vi "Avoid Obstacle with Unicycle Model.vi"(9 "V forward":dbl, 10 "Posture In":dbl[](array[numeric]), 11 "IF readings\n(meters)":dbl[](array[numeric]) format="%_6g") -> (3 "Frame Velocity":dbl[](array[numeric]))   [LabVIEW 2016]
uses:
  <vilib>/Analysis/coordinate.llb/Angle Range (Degree).ctl
  <vilib>/Analysis/coordinate.llb/Angle Units.ctl
  <vilib>/Analysis/coordinate.llb/Wrap Angle (scalar).vi
  <vilib>/Analysis/NI_AAL_Angle.lvlib
panel:
  in  "K Gain":dbl=12.0
  out "atan2(y,x)":dbl
  out "x-y":dbl
  out "output":dbl format="%.2f"
  in  "Sensor Gain":dbl[](array[numeric])=[1.0, 1.0, 0.5, 1.0, 1.0]
  out "ir distances wf":dbl[][](array[numeric])
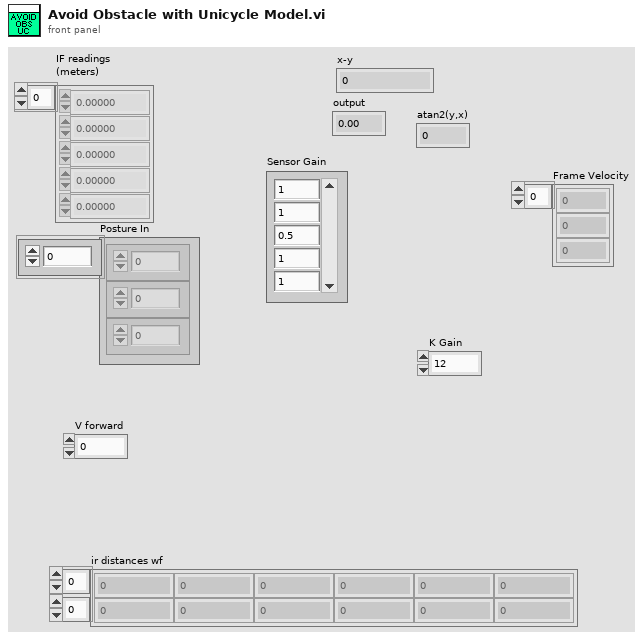
[diagram p1: front panel]
types:
  T1 = typedef "NI_AAL_Angle.lvlib/Angle Units.ctl" = i32
  T2 = typedef "NI_AAL_Angle.lvlib/Angle Range (Degree).ctl" = u16
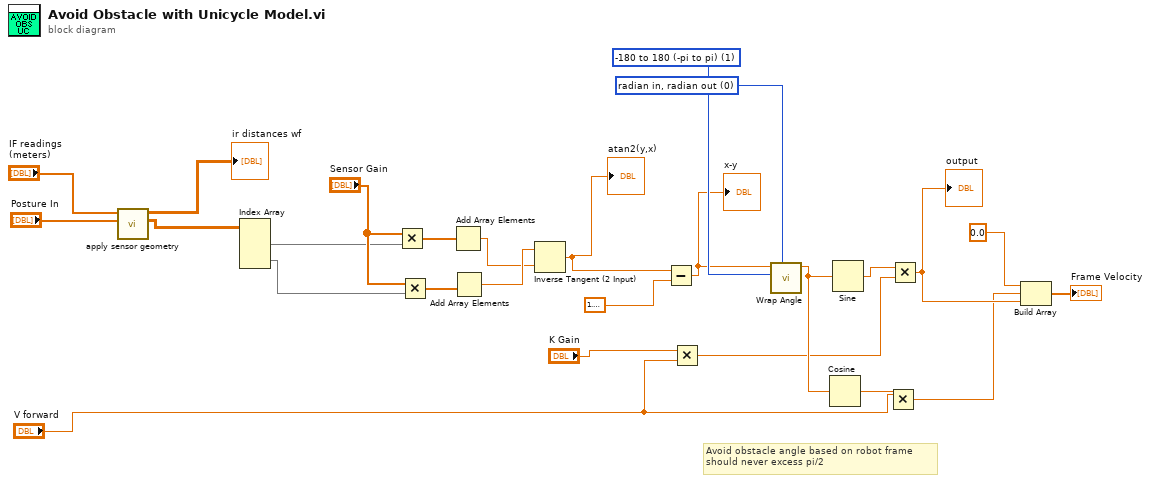
[diagram p0: block diagram]
diagram:
  w16 = T1 0 items=["radian in, radian out", "radian in, degree out", "degree in, degree out", "degree in, radian out"] ("angle units")
  w17 = T2 1 items=["none", "-180 to 180 (-pi to pi)", "0 to 360 (0 to 2pi)"] ("angle range")
  # "Avoid obstacle angle based on robot frame \nshould never excess pi/2"
  n1 = call "apply sensor geometry.vi"("Posture In"="Posture In", "IF readings\n(meters)"="IF readings\n(meters)") -> ("ir distances rf"=w13:dbl[][], "ir distances wf"=→"ir distances wf":dbl[][])  [unwired: 8 in]
  n2 = Index Array(array=w13) -> (element #1=w12:dbl[], element #2=w11:dbl[])  [unwired: 4 in]
  n3 = Multiply(x="Sensor Gain", y=w12) -> (x*y=w22:dbl[])
  n4 = Multiply(x="Sensor Gain", y=w11) -> (x*y=w21:dbl[])
  n5 = Add Array Elements(numeric array=w22) -> (sum=w19:dbl)
  n6 = Add Array Elements(numeric array=w21) -> (sum=w20:dbl)
  n7 = Inverse Tangent (2 Input)(1:w19, 2:w20) -> (0:w18:dbl)
  "atan2(y,x)" <- w18
  n8 = Subtract(x=w18, y=1.5707963267948966) -> (x-y=w7:dbl)
  "x-y" <- w7
  n9 = Multiply(x="K Gain", y="V forward") -> (x*y=w3:dbl)
  n10 = call-poly <vilib>:"Wrap Angle.vi"("angle units"=w16, "angle range"=w17, "angle in"=w7) -> ("angle out"=w6:dbl)  [unwired: 7 in, 1 out]
  n11 = Cosine(x=w6) -> (cos(x)=w5:dbl)
  n12 = Sine(x=w6) -> (sin(x)=w9:dbl)
  n13 = Multiply(x="V forward", y=w5) -> (x*y=w4:dbl)
  n14 = Multiply(x=w9, y=w3) -> (x*y=w8:dbl)
  "output" <- w8
  n15 = Build Array(0.0 ("element"), w4, w8) -> (→"Frame Velocity":dbl[])
